vi "Append New Table (Double).vi"(4 "Row.Headers":string[](array[string]), 6 "Column.Headers":string[](array[string]), 8 "error in (no error)":errorcluster, 9 "Cell.Style":refnum<class "Style.lvclass">, 10 "Table.Data":dbl[][](array[numeric]), 11 "xwpfDocument in":refnum<class "xwpfDocument.lvclass">) -> (0 "error out":errorcluster, 3 "xwpfDocument out":refnum<class "xwpfDocument.lvclass">)   [LabVIEW 2017]
uses:
  xwpfTable/xwpfTable.lvclass
  xwpfDocument.lvclass
  C:/Users/Neo/Desktop/Dev_Tools_BR/LabVIEW_NPOI/src/lib/NPOI 2.1.1/NPOI.OOXML.dll
  lib/NPOI 2.1.1/NPOI.OOXML.dll
  C:/Users/Neo/Desktop/Dev_Tools_BR/LabVIEW_NPOI/src/LabVIEW NPOI/xwpfDocument.Element/xwpfDocument.Element.lvclass
  Styles/Style/Style.lvclass
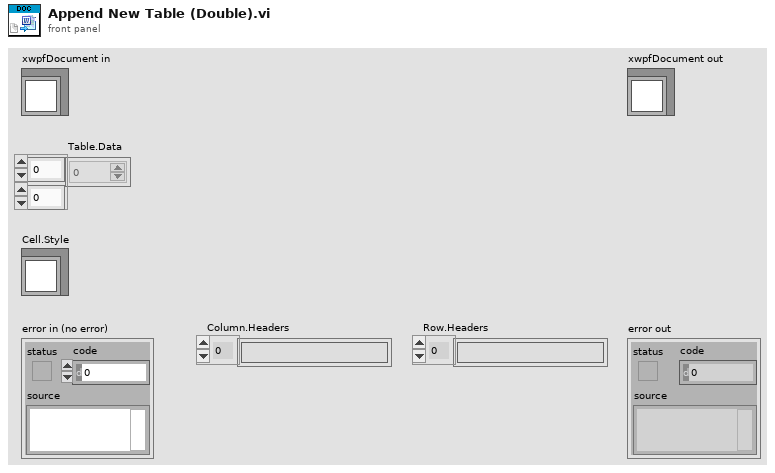
[diagram p1: front panel]
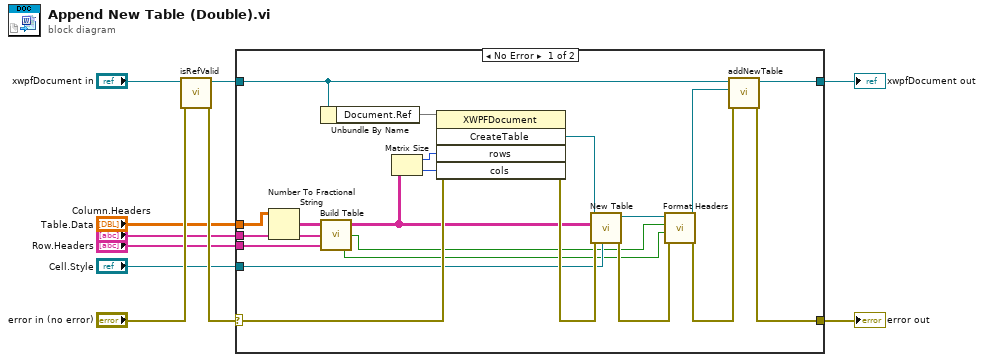
[diagram p0: block diagram]
diagram:
  n1 = call-dynamic "isRefValid.vi"("error in (no error)"="error in (no error)", "xwpfDocument in"="xwpfDocument in") -> ("error out"=w5:errorcluster, "xwpfDocument out"=w7:refnum<class "xwpfDocument.lvclass">)  [unwired: 8 in]
  n2 = case shown="No Error" w5 {
    selector: w5 -> [w26 w33]
    tunnel: [w30 w33] -> w10
    tunnel: [w31 w32] -> w8
    tunnel: w7 -> [w29 w32]
    tunnel: "Table.Data" -> [w12 _]
    tunnel: "Cell.Style" -> [w19 _]
    tunnel: "Row.Headers" -> [w21 _]
    tunnel: "Column.Headers" -> [w20 _]
    frame No Error {
      n3 = Number To Fractional String(number=w12) -> (F-format string=w11:string[][])  [unwired: 3 in]
      n4 = Unbundle By Name(w29) -> ("Document.Ref"=w27)
      n5 = call "Build Table.vi"("Row.Headers"=w21, "Column.Headers"=w20, "Table.Data.Text"=w11) -> ("Column.Headers"=w13:bool, "Row.Headers"=w14:bool, "Table.Text"=w22:string[][])
      n6 = Matrix Size(0:w22) -> (1:w25:i32, 2:w24:i32)
      n7 = invoke class="XWPFDocument" method="CreateTable"(reference=w27, error in=w26, "rows"=w25, "cols"=w24) -> (error out=w28:errorcluster, "CreateTable"=w23:refnum<k24>)  [unwired: 1 in, 3 out]
      n8 = call "New Table.vi"("Cell.Style"=w19, "error in (no error)"=w28, "Table"=w22, "Table Ref"=w23) -> ("error out"=w16:errorcluster, "xwpfTable out"=w18:refnum<class "xwpfTable.lvclass">)  [unwired: 6 in]
      n9 = call "Format Headers.vi"("error in (no error)"=w16, "Column.Headers"=w13, "Row.Headers"=w14, "xwpfTable in"=w18) -> ("error out"=w15:errorcluster, "xwpfTable out"=w17:refnum<class "xwpfTable.lvclass">)  [unwired: 6 in]
      n10 = call "addNewTable.vi"("error in (no error)"=w15, "New Paragraph"=w17, "xwpfDocument in"=w29) -> ("error out"=w30:errorcluster, "xwpfDocument out"=w31:refnum<class "xwpfDocument.lvclass">)  [unwired: 7 in]
    }
    frame Error {
    }
  }
  "error out" <- w10
  "xwpfDocument out" <- w8
